vi "OFDM_SuperpositionedBitDetect_SIC.vi"(0 "Input symbols":cdb[](array[numeric]) format="%.2f", 1 "Modulation type":T1(ring), 3 "error in (no error)":errorcluster) -> (5 "Base Bits":i8[](array[numeric]), 6 "SC Symbols":cdb[](array[numeric]), 7 "SC Bits":i8[](array[numeric]), 10 "error out":errorcluster)   [LabVIEW 2022 SP3]
uses:
  <vilib>/addons/Modulation/Digital/General/MT Map QAM Symbols to Bits.vi
  <vilib>/addons/Modulation/Digital/General/MT Map Bits to QAM Symbols.vi
  <vilib>/addons/Modulation/Digital/General/MT Map PSK Symbols to Bits.vi
  <vilib>/addons/Modulation/Digital/General/MT Map Bits to PSK Symbols.vi
  <vilib>/addons/Modulation/niDMT.lvlib
panel:
  in  "Point scaler":dbl(slide)=0.9662650602409638 scale=0.8..1.2
  in  "Slide":dbl(slide)=4.5 step=0.1 scale=0.0..10.0
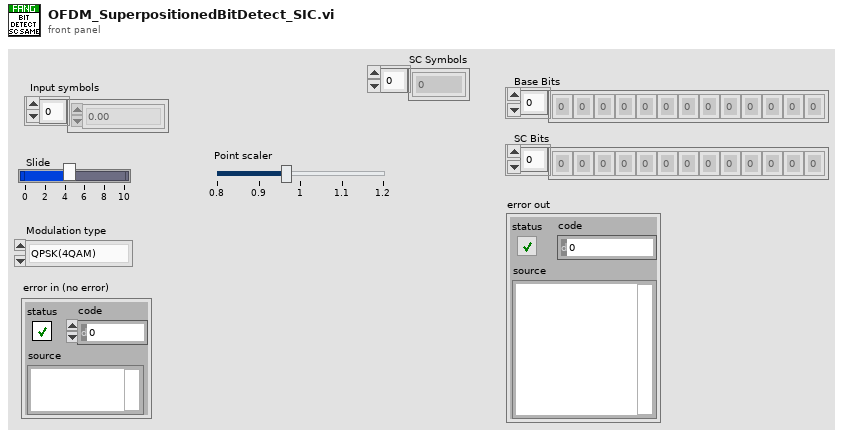
[diagram p1: front panel]
types:
  T1 = enum16{"QPSK(4QAM)", "64QAM", "16QAM", "BPSK", "BPSK Vertical"}
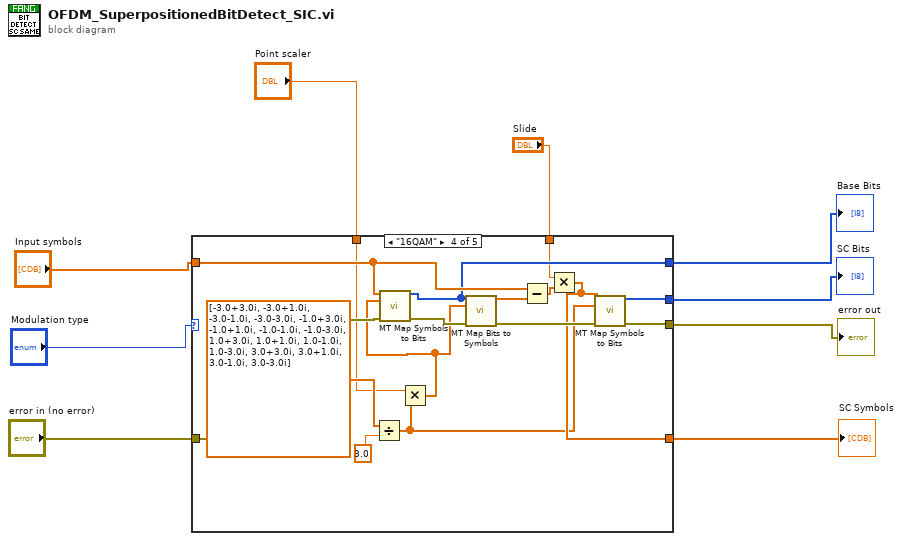
[diagram p0: block diagram]
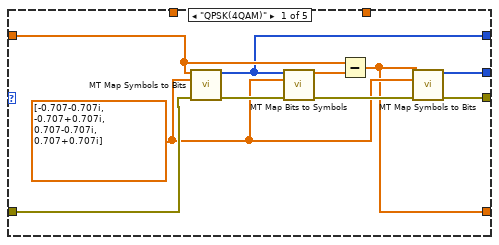
[diagram p2: hidden frame]
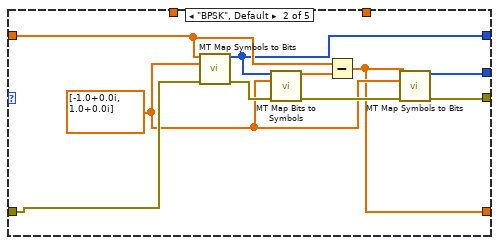
[diagram p3: hidden frame]
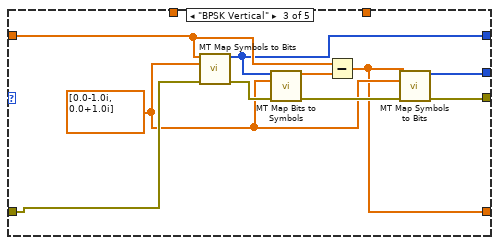
[diagram p4: hidden frame]
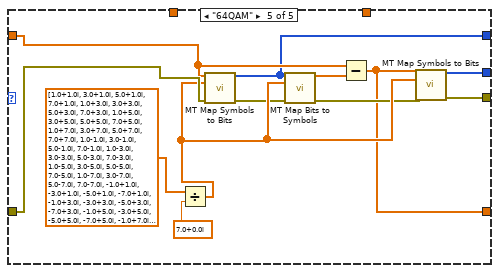
[diagram p5: hidden frame]
diagram:
  n1 = case shown="\"16QAM\"" "Modulation type" {
    tunnel: "Input symbols" -> [w16 w22 w32 w49 w62]
    tunnel: "error in (no error)" -> [w19 w29 w39 w55 w65]
    tunnel: [w12 w25 w35 w52 w61] -> w6
    tunnel: [w14 w26 w36 w51 w60] -> w5
    tunnel: [w11 w21 w31 w46 w57] -> w4
    tunnel: [w10 w20 w30 w44 w56] -> w3
    tunnel: "Point scaler" -> [_ _ _ w42 _]
    tunnel: "Slide" -> [_ _ _ w40 _]
    frame "QPSK(4QAM)" {
      w13 = cdb[] [-0.707-0.707i, -0.707+0.707i, 0.707-0.707i, 0.707+0.707i] ("symbol map")
      n2 = call-poly <vilib>:"MT Map Symbols to Bits.vi"("symbols"=w16, "symbol map"=w13, "error in (no error)"=w19) -> ("output bit stream"=w11:i8[], "error out"=w18:errorcluster)  [unwired: 11 in]
      n3 = call-poly <vilib>:"MT Map Bits to Symbols.vi"("input bit stream"=w11, "symbol map"=w13, "error in (no error)"=w18) -> ("symbols"=w17:cdb[], "error out"=w15:errorcluster)  [unwired: 11 in]
      n4 = Subtract(x=w16, y=w17) -> (x-y=w10:cdb[])
      n5 = call-poly <vilib>:"MT Map Symbols to Bits.vi"("symbols"=w10, "symbol map"=w13, "error in (no error)"=w15) -> ("output bit stream"=w12:i8[], "error out"=w14:errorcluster)  [unwired: 11 in]
    }
    frame "BPSK", Default {
      w24 = cdb[] [-1.0+0.0i, 1.0+0.0i] ("symbol map")
      n6 = call-poly <vilib>:"MT Map Symbols to Bits.vi"("symbols"=w22, "symbol map"=w24, "error in (no error)"=w29) -> ("output bit stream"=w21:i8[], "error out"=w28:errorcluster)  [unwired: 11 in]
      n7 = call-poly <vilib>:"MT Map Bits to Symbols.vi"("input bit stream"=w21, "symbol map"=w24, "error in (no error)"=w28) -> ("symbols"=w23:cdb[], "error out"=w27:errorcluster)  [unwired: 11 in]
      n8 = Subtract(x=w22, y=w23) -> (x-y=w20:cdb[])
      n9 = call-poly <vilib>:"MT Map Symbols to Bits.vi"("symbols"=w20, "symbol map"=w24, "error in (no error)"=w27) -> ("output bit stream"=w25:i8[], "error out"=w26:errorcluster)  [unwired: 11 in]
    }
    frame "BPSK Vertical" {
      w34 = cdb[] [0.0-1.0i, 0.0+1.0i] ("symbol map")
      n10 = call-poly <vilib>:"MT Map Symbols to Bits.vi"("symbols"=w32, "symbol map"=w34, "error in (no error)"=w39) -> ("output bit stream"=w31:i8[], "error out"=w38:errorcluster)  [unwired: 11 in]
      n11 = call-poly <vilib>:"MT Map Bits to Symbols.vi"("input bit stream"=w31, "symbol map"=w34, "error in (no error)"=w38) -> ("symbols"=w33:cdb[], "error out"=w37:errorcluster)  [unwired: 11 in]
      n12 = Subtract(x=w32, y=w33) -> (x-y=w30:cdb[])
      n13 = call-poly <vilib>:"MT Map Symbols to Bits.vi"("symbols"=w30, "symbol map"=w34, "error in (no error)"=w37) -> ("output bit stream"=w35:i8[], "error out"=w36:errorcluster)  [unwired: 11 in]
    }
    frame "16QAM" {
      n14 = Divide(x=cdb[] [-3.0+3.0i, -3.0+1.0i, -3.0-1.0i, -3.0-3.0i, -1.0+3.0i, -1.0+1.0i, -1.0-1.0i, -1.0-3.0i, 1.0+3.0i, 1.0+1.0i, 1.0-1.0i, 1.0-3.0i, 3.0+3.0i, 3.0+1.0i, 3.0-1.0i, 3.0-3.0i] ("symbol map"), y=3.0) -> (x/y=w43:cdb[])
      n15 = Multiply(x=w42, y=w43) -> (x*y=w41:cdb[])
      n16 = call-poly <vilib>:"MT Map Symbols to Bits.vi"("symbols"=w49, "symbol map"=w41, "error in (no error)"=w55) -> ("output bit stream"=w46:i8[], "error out"=w48:errorcluster)  [unwired: 11 in]
      n17 = call-poly <vilib>:"MT Map Bits to Symbols.vi"("input bit stream"=w46, "symbol map"=w41, "error in (no error)"=w48) -> ("symbols"=w50:cdb[], "error out"=w47:errorcluster)  [unwired: 11 in]
      n18 = Subtract(x=w49, y=w50) -> (x-y=w45:cdb[])
      n19 = Multiply(x=w40, y=w45) -> (x*y=w44:cdb[])
      n20 = call-poly <vilib>:"MT Map Symbols to Bits.vi"("symbols"=w44, "symbol map"=w43, "error in (no error)"=w47) -> ("output bit stream"=w52:i8[], "error out"=w51:errorcluster)  [unwired: 11 in]
    }
    frame "64QAM" {
      n21 = Divide(x=cdb[] [1.0+1.0i, 3.0+1.0i, 5.0+1.0i, 7.0+1.0i, 1.0+3.0i, 3.0+3.0i, 5.0+3.0i, 7.0+3.0i, 1.0+5.0i, 3.0+5.0i, 5.0+5.0i, 7.0+5.0i, 1.0+7.0i, 3.0+7.0i, 5.0+7.0i, 7.0+7.0i, 1.0-1.0i, 3.0-1.0i, 5.0-1.0i, 7.0-1.0i, 1.0-3.0i, 3.0-3.0i, 5.0-3.0i, 7.0-3.0i, 1.0-5.0i, 3.0-5.0i, 5.0-5.0i, 7.0-5.0i, 1.0-7.0i, 3.0-7.0i, 5.0-7.0i, 7.0-7.0i, -1.0+1.0i, -3.0+1.0i, -5.0+1.0i, -7.0+1.0i, -1.0+3.0i, -3.0+3.0i, -5.0+3.0i, -7.0+3.0i, -1.0+5.0i, -3.0+5.0i, -5.0+5.0i, -7.0+5.0i, -1.0+7.0i, -3.0+7.0i, -5.0+7.0i, -7.0+7.0i, -1.0-1.0i, -3.0-1.0i, -5.0-1.0i, -7.0-1.0i, -1.0-3.0i, -3.0-3.0i, -5.0-3.0i, -7.0-3.0i, -1.0-5.0i, -3.0-5.0i, -5.0-5.0i, -7.0-5.0i, -1.0-7.0i, -3.0-7.0i, -5.0-7.0i, -7.0-7.0i] ("appended array"), y=cdb 7.0+0.0i) -> (x/y=w64:cdb[])
      n22 = call-poly <vilib>:"MT Map Symbols to Bits.vi"("symbols"=w62, "symbol map"=w64, "error in (no error)"=w65) -> ("output bit stream"=w57:i8[], "error out"=w59:errorcluster)  [unwired: 11 in]
      n23 = call-poly <vilib>:"MT Map Bits to Symbols.vi"("input bit stream"=w57, "symbol map"=w64, "error in (no error)"=w59) -> ("symbols"=w63:cdb[], "error out"=w58:errorcluster)  [unwired: 11 in]
      n24 = Subtract(x=w62, y=w63) -> (x-y=w56:cdb[])
      n25 = call-poly <vilib>:"MT Map Symbols to Bits.vi"("symbols"=w56, "symbol map"=w64, "error in (no error)"=w58) -> ("output bit stream"=w61:i8[], "error out"=w60:errorcluster)  [unwired: 11 in]
    }
  }
  "SC Bits" <- w6
  "error out" <- w5
  "Base Bits" <- w4
  "SC Symbols" <- w3
